vi "Save Cfg to GXML.vi"(8 "error in":errorcluster, 11 "Chassis Cfg":refnum<class "ChassisCfg.lvclass">) -> (0 "error out":errorcluster, 2 "GXML String":string="<GXML_Root>\r\n  <VoltGroup mems='3' id='Static Voltages'>\r\n    <GroupName type='String'>Static Voltages</GroupName>\r\n    <MeasType type='Enum U16' sel='Voltage'>0</MeasType>\r\n    <GroupMems dim='[33]' type='Cluster'>\r\n      <VoltChan mems='2'>\r\n        <ChanHdr mems='5'>\r\n          <ChanName type='String'>Mod4/ai0</ChanName>\r\n          <Alias type='String'></Alias>\r\n          <ModbusAddr type='String'>300047</ModbusAddr>\r\n          <Device type='String'>NI 9205</Device>\r\n          <ToModBus type='Bool'>TRUE</ToModBus>\r\n        </ChanHdr>\r\n        <VoltChanCfg mems='3'>\r\n          <VRange type='DBL'>10</VRange>\r\n          <Term_Cfg type='U16'>10083</Term_Cfg>\r\n          <Coupling type='U16'>10050</Coupling>\r\n        </VoltChanCfg>\r\n      </VoltChan>\r\n      <VoltChan mems='2'>\r\n        <ChanHdr mems='5'>\r\n          <ChanName type='String'>Mod4/ai1</ChanName>\r\n          <Alias type='String'></Alias>\r\n          <ModbusAddr type='String'>300049</ModbusAddr>\r\n          <Device type='String'>NI 9205</Device>\r\n          <ToModBus type='Bool'>TRUE</ToModBus>\r\n        </ChanHdr>\r\n        <VoltChanCfg mems='3'>\r\n          <VRange type='DBL'>10</VRange>\r\n          <Term_Cfg type='U16'>10083</Term_Cfg>\r\n          <Coupling type='U16'>10050</Coupling>\r\n        </VoltChanCfg>\r\n      </VoltChan>\r\n      <VoltChan mems='2'>\r\n        <ChanHdr mems='5'>\r\n          <ChanName type='String'>Mod4/ai2</ChanName>\r\n          <Alias type='String'></Alias>\r\n          <ModbusAddr type='String'>300051</ModbusAddr>\r\n          <Device type='String'>NI 9205</Device>\r\n          <ToModBus type='Bool'>TRUE</ToModBus>\r\n        </ChanHdr>\r\n        <VoltChanCfg mems='3'>\r\n          <VRange type='DBL'>10</VRange>\r\n          <Term_Cfg type='U16'>10083</Term_Cfg>\r\n          <Coupling type='U16'>10050</Coupling>\r\n        </VoltChanCfg>\r\n      </VoltChan>\r\n      <VoltChan mems='2'>\r\n        <ChanHdr mems='5'>\r\n          <ChanName type='String'>Mod4/ai3</ChanName>\r\n          <Alias type='String'></Alias>\r\n          <ModbusAddr type='String'>300053</ModbusAddr>\r\n          <Device type='String'>NI 9205</Device>\r\n          <ToModBus type='Bool'>TRUE</ToModBus>\r\n        </ChanHdr>\r\n        <VoltChanCfg mems='3'>\r\n          <VRange type='DBL'>10</VRange>\r\n          <Term_Cfg type='U16'>10083</Term_Cfg>\r\n          <Coupling type='U16'>10050</Coupling>\r\n        </VoltChanCfg>\r\n      </VoltChan>\r\n      <VoltChan mems='2'>\r\n        <ChanHdr mems='5'>\r\n          <ChanName type='String'>Mod4/ai4</ChanName>\r\n          <Alias type='String'></Alias>\r\n          <ModbusAddr type='String'>300055</ModbusAddr>\r\n          <Device type='String'>NI 9205</Device>\r\n          <ToModBus type='Bool'>TRUE</ToModBus>\r\n        </ChanHdr>\r\n        <VoltChanCfg mems='3'>\r\n          <VRange type='DBL'>10</VRange>\r\n          <Term_Cfg type='U16'>10083</Term_Cfg>\r\n          <Coupling type='U16'>10050</Coupling>\r\n        </VoltChanCfg>\r\n      </VoltChan>\r\n      <VoltChan mems='2'>\r\n        <ChanHdr mems='5'>\r\n          <ChanName type='String'>Mod4/ai5</ChanName>\r\n          <Alias type='String'></Alias>\r\n          <ModbusAddr type='String'>300057</ModbusAddr>\r\n          <Device type='String'>NI 9205</Device>\r\n          <ToModBus type='Bool'>TRUE</ToModBus>\r\n        </ChanHdr>\r\n        <VoltChanCfg mems='3'>\r\n          <VRange type='DBL'>10</VRange>\r\n          <Term_Cfg type='U16'>10083</Term_Cfg>\r\n          <Coupling type='U16'>10050</Coupling>\r\n        </VoltChanCfg>\r\n      </VoltChan>\r\n      <VoltChan mems='2'>\r\n        <ChanHdr mems='5'>\r\n          <ChanName type='String'>Mod4/ai6</ChanName>\r\n          <Alias type='String'></Alias>\r\n          <ModbusAddr type='String'>300059</ModbusAddr>\r\n          <Device type='String'>NI 9205</Device>\r\n          <ToModBus type='Bool'>TRUE</ToModBus>\r\n        </ChanHdr>\r\n        <VoltChanCfg mems='3'>\r\n          <VRange type='DBL'>10</VRange>\r\n          <Term_Cfg type='U16'>10083</Term_Cfg>\r\n          <Coupling type='U16'>10050</Coupling>\r\n        </VoltChanCfg>\r\n      </VoltChan>\r\n      <VoltChan mems='2'>\r\n        <ChanHdr mems='5'>\r\n          <ChanName type='String'>Mod4/ai7</ChanName>\r\n          <Alias type='String'></Alias>\r\n          <ModbusAddr type='String'>300061</ModbusAddr>\r\n          <Device type='String'>NI 9205</Device>\r\n          <ToModBus type='Bool'>TRUE</ToModBus>\r\n        </ChanHdr>\r\n        <VoltChanCfg mems='3'>\r\n          <VRange type='DBL'>10</VRange>\r\n          <Term_Cfg type='U16'>10083</Term_Cfg>\r\n          <Coupling type='U16'>10050</Coupling>\r\n        </VoltChanCfg>\r\n      </VoltChan>\r\n      <VoltChan mems='2'>\r\n        <ChanHdr mems='5'>\r\n          <ChanName type='String'>Mod4/ai8</ChanName>\r\n          <Alias type='String'></Alias>\r\n          <ModbusAddr type='String'>300063</ModbusAddr>\r\n          <Device type='String'>NI 9205</Device>\r\n          <ToModBus type='Bool'>TRUE</ToModBus>\r\n        </ChanHdr>\r\n        <VoltChanCfg mems='3'>\r\n          <VRange type='DBL'>10</VRange>\r\n          <Term_Cfg type='U16'>10083</Term_Cfg>\r\n          <Coupling type='U16'>10050</Coupling>\r\n        </VoltChanCfg>\r\n      </VoltChan>\r\n      <VoltChan mems='2'>\r\n        <ChanHdr mems='5'>\r\n          <ChanName type='String'>Mod4/ai9</ChanName>\r\n          <Alias type='String'></Alias>\r\n          <ModbusAddr type='String'>300065</ModbusAddr>\r\n          <Device type='String'>NI 9205</Device>\r\n          <ToModBus type='Bool'>TRUE</ToModBus>\r\n        </ChanHdr>\r\n        <VoltChanCfg mems='3'>\r\n          <VRange type='DBL'>10</VRange>\r\n          <Term_Cfg type='U16'>10083</Term_Cfg>\r\n          <Coupling type='U16'>10050</Coupling>\r\n        </VoltChanCfg>\r\n      </VoltChan>\r\n      <VoltChan mems='2'>\r\n        <ChanHdr mems='5'>\r\n          <ChanName type='String'>Mod4/ai10</ChanName>\r\n          <Alias type='String'></Alias>\r\n          <ModbusAddr type='String'>300067</ModbusAddr>\r\n          <Device type='String'>NI 9205</Device>\r\n          <ToModBus type='Bool'>TRUE</ToModBus>\r\n        </ChanHdr>\r\n        <VoltChanCfg mems='3'>\r\n          <VRange type='DBL'>10</VRange>\r\n          <Term_Cfg type='U16'>10083</Term_Cfg>\r\n          <Coupling type='U16'>10050</Coupling>\r\n        </VoltChanCfg>\r\n      </VoltChan>\r\n      <VoltChan mems='2'>\r\n        <ChanHdr mems='5'>\r\n          <ChanName type='String'>Mod4/ai11</ChanName>\r\n          <Alias type='String'></Alias>\r\n          <ModbusAddr type='String'>300069</ModbusAddr>\r\n          <Device type='String'>NI 9205</Device>\r\n          <ToModBus type='Bool'>TRUE</ToModBus>\r\n        </ChanHdr>\r\n        <VoltChanCfg mems='3'>\r\n          <VRange type='DBL'>10</VRange>\r\n          <Term_Cfg type='U16'>10083</Term_Cfg>\r\n          <Coupling type='U16'>10050</Coupling>\r\n        </VoltChanCfg>\r\n      </VoltChan>\r\n      <VoltChan mems='2'>\r\n        <ChanHdr mems='5'>\r\n          <ChanName type='String'>Mod4/ai12</ChanName>\r\n          <Alias type='String'></Alias>\r\n          <ModbusAddr type='String'>300071</ModbusAddr>\r\n          <Device type='String'>NI 9205</Device>\r\n          <ToModBus type='Bool'>TRUE</ToModBus>\r\n        </ChanHdr>\r\n        <VoltChanCfg mems='3'>\r\n          <VRange type='DBL'>10</VRange>\r\n          <Term_Cfg type='U16'>10083</Term_Cfg>\r\n          <Coupling type='U16'>10050</Coupling>\r\n        </VoltChanCfg>\r\n      </VoltChan>\r\n      <VoltChan mems='2'>\r\n        <ChanHdr mems='5'>\r\n          <ChanName type='String'>Mod4/ai13</ChanName>\r\n          <Alias type='String'></Alias>\r\n          <ModbusAddr type='String'>300073</ModbusAddr>\r\n          <Device type='String'>NI 9205</Device>\r\n          <ToModBus type='Bool'>TRUE</ToModBus>\r\n        </ChanHdr>\r\n        <VoltChanCfg mems='3'>\r\n          <VRange type='DBL'>10</VRange>\r\n          <Term_Cfg type='U16'>10083</Term_Cfg>\r\n          <Coupling type='U16'>10050</Coupling>\r\n        </VoltChanCfg>\r\n      </VoltChan>\r\n      <VoltChan mems='2'>\r\n        <ChanHdr mems='5'>\r\n          <ChanName type='String'>Mod4/ai14</ChanName>\r\n          <Alias type='String'></Alias>\r\n          <ModbusAddr type='String'>300075</ModbusAddr>\r\n          <Device type='String'>NI 9205</Device>\r\n          <ToModBus type='Bool'>TRUE</ToModBus>\r\n        </ChanHdr>\r\n        <VoltChanCfg mems='3'>\r\n          <VRange type='DBL'>10</VRange>\r\n          <Term_Cfg type='U16'>10083</Term_Cfg>\r\n          <Coupling type='U16'>10050</Coupling>\r\n        </VoltChanCfg>\r\n      </VoltChan>\r\n      <VoltChan mems='2'>\r\n        <ChanHdr mems='5'>\r\n          <ChanName type='String'>Mod4/ai15</ChanName>\r\n          <Alias type='String'></Alias>\r\n          <ModbusAddr type='String'>300077</ModbusAddr>\r\n          <Device type='String'>NI 9205</Device>\r\n          <ToModBus type='Bool'>TRUE</ToModBus>\r\n        </ChanHdr>\r\n        <VoltChanCfg mems='3'>\r\n          <VRange type='DBL'>10</VRange>\r\n          <Term_Cfg type='U16'>10083</Term_Cfg>\r\n          <Coupling type='U16'>10050</Coupling>\r\n        </VoltChanCfg>\r\n      </VoltChan>\r\n      <VoltChan mems='2'>\r\n        <ChanHdr mems='5'>\r\n          <ChanName type='String'>Mod4/ai16</ChanName>\r\n          <Alias type='String'></Alias>\r\n          <ModbusAddr type='String'>300079</ModbusAddr>\r\n          <Device type='String'>NI 9205</Device>\r\n          <ToModBus type='Bool'>TRUE</ToModBus>\r\n        </ChanHdr>\r\n        <VoltChanCfg mems='3'>\r\n          <VRange type='DBL'>10</VRange>\r\n          <Term_Cfg type='U16'>10083</Term_Cfg>\r\n          <Coupling type='U16'>10050</Coupling>\r\n        </VoltChanCfg>\r\n      </VoltChan>\r\n      <VoltChan mems='2'>\r\n        <ChanHdr mems='5'>\r\n          <ChanName type='String'>Mod4/ai17</ChanName>\r\n          <Alias type='String'></Alias>\r\n          <ModbusAddr type='String'>300081</ModbusAddr>\r\n          <Device type='String'>NI 9205</Device>\r\n          <ToModBus type='Bool'>TRUE</ToModBus>\r\n        </ChanHdr>\r\n        <VoltChanCfg mems='3'>\r\n          <VRange type='DBL'>10</VRange>\r\n          <Term_Cfg type='U16'>10083</Term_Cfg>\r\n          <Coupling type='U16'>10050</Coupling>\r\n        </VoltChanCfg>\r\n      </VoltChan>\r\n      <VoltChan mems='2'>\r\n        <ChanHdr mems='5'>\r\n          <ChanName type='String'>Mod4/ai18</ChanName>\r\n          <Alias type='String'></Alias>\r\n          <ModbusAddr type='String'>300083</ModbusAddr>\r\n          <Device type='String'>NI 9205</Device>\r\n          <ToModBus type='Bool'>TRUE</ToModBus>\r\n        </ChanHdr>\r\n        <VoltChanCfg mems='3'>\r\n          <VRange type='DBL'>10</VRange>\r\n          <Term_Cfg type='U16'>10083</Term_Cfg>\r\n          <Coupling type='U16'>10050</Coupling>\r\n        </VoltChanCfg>\r\n      </VoltChan>\r\n      <VoltChan mems='2'>\r\n        <ChanHdr mems='5'>\r\n          <ChanName type='String'>Mod4/ai19</ChanName>\r\n          <Alias type='String'></Alias>\r\n          <ModbusAddr type='String'>300085</ModbusAddr>\r\n          <Device type='String'>NI 9205</Device>\r\n          <ToModBus type='Bool'>TRUE</ToModBus>\r\n        </ChanHdr>\r\n        <VoltChanCfg mems='3'>\r\n          <VRange type='DBL'>10</VRange>\r\n          <Term_Cfg type='U16'>10083</Term_Cfg>\r\n          <Coupling type='U16'>10050</Coupling>\r\n        </VoltChanCfg>\r\n      </VoltChan>\r\n      <VoltChan mems='2'>\r\n        <ChanHdr mems='5'>\r\n          <ChanName type='String'>Mod4/ai20</ChanName>\r\n          <Alias type='String'></Alias>\r\n          <ModbusAddr type='String'>300087</ModbusAddr>\r\n          <Device type='String'>NI 9205</Device>\r\n          <ToModBus type='Bool'>TRUE</ToModBus>\r\n        </ChanHdr>\r\n        <VoltChanCfg mems='3'>\r\n          <VRange type='DBL'>10</VRange>\r\n          <Term_Cfg type='U16'>10083</Term_Cfg>\r\n          <Coupling type='U16'>10050</Coupling>\r\n        </VoltChanCfg>\r\n      </VoltChan>\r\n      <VoltChan mems='2'>\r\n        <ChanHdr mems='5'>\r\n          <ChanName type='String'>Mod4/ai21</ChanName>\r\n          <Alias type='String'></Alias>\r\n          <ModbusAddr type='String'>300089</ModbusAddr>\r\n          <Device type='String'>NI 9205</Device>\r\n          <ToModBus type='Bool'>TRUE</ToModBus>\r\n        </ChanHdr>\r\n        <VoltChanCfg mems='3'>\r\n          <VRange type='DBL'>10</VRange>\r\n          <Term_Cfg type='U16'>10083</Term_Cfg>\r\n          <Coupling type='U16'>10050</Coupling>\r\n        </VoltChanCfg>\r\n      </VoltChan>\r\n      <VoltChan mems='2'>\r\n        <ChanHdr mems='5'>\r\n          <ChanName type='String'>Mod4/ai22</ChanName>\r\n          <Alias type='String'></Alias>\r\n          <ModbusAddr type='String'>300091</ModbusAddr>\r\n          <Device type='String'>NI 9205</Device>\r\n          <ToModBus type='Bool'>TRUE</ToModBus>\r\n        </ChanHdr>\r\n        <VoltChanCfg mems='3'>\r\n          <VRange type='DBL'>10</VRange>\r\n          <Term_Cfg type='U16'>10083</Term_Cfg>\r\n          <Coupling type='U16'>10050</Coupling>\r\n        </VoltChanCfg>\r\n      </VoltChan>\r\n      <VoltChan mems='2'>\r\n        <ChanHdr mems='5'>\r\n          <ChanName type='String'>Mod4/ai23</ChanName>\r\n          <Alias type='String'></Alias>\r\n          <ModbusAddr type='String'>300093</ModbusAddr>\r\n          <Device type='String'>NI 9205</Device>\r\n          <ToModBus type='Bool'>TRUE</ToModBus>\r\n        </ChanHdr>\r\n        <VoltChanCfg mems='3'>\r\n          <VRange type='DBL'>10</VRange>\r\n          <Term_Cfg type='U16'>10083</Term_Cfg>\r\n          <Coupling type='U16'>10050</Coupling>\r\n        </VoltChanCfg>\r\n      </VoltChan>\r\n      <VoltChan mems='2'>\r\n        <ChanHdr mems='5'>\r\n          <ChanName type='String'>Mod4/ai24</ChanName>\r\n          <Alias type='String'></Alias>\r\n          <ModbusAddr type='String'>300095</ModbusAddr>\r\n          <Device type='String'>NI 9205</Device>\r\n          <ToModBus type='Bool'>TRUE</ToModBus>\r\n        </ChanHdr>\r\n        <VoltChanCfg mems='3'>\r\n          <VRange type='DBL'>10</VRange>\r\n          <Term_Cfg type='U16'>10083</Term_Cfg>\r\n          <Coupling type='U16'>10050</Coupling>\r\n        </VoltChanCfg>\r\n      </VoltChan>\r\n      <VoltChan mems='2'>\r\n        <ChanHdr mems='5'>\r\n          <ChanName type='String'>Mod4/ai25</ChanName>\r\n          <Alias type='String'></Alias>\r\n          <ModbusAddr type='String'>300097</ModbusAddr>\r\n          <Device type='String'>NI 9205</Device>\r\n          <ToModBus type='Bool'>TRUE</ToModBus>\r\n        </ChanHdr>\r\n        <VoltChanCfg mems='3'>\r\n          <VRange type='DBL'>10</VRange>\r\n          <Term_Cfg type='U16'>10083</Term_Cfg>\r\n          <Coupling type='U16'>10050</Coupling>\r\n        </VoltChanCfg>\r\n      </VoltChan>\r\n      <VoltChan mems='2'>\r\n        <ChanHdr mems='5'>\r\n          <ChanName type='String'>Mod4/ai26</ChanName>\r\n          <Alias type='String'></Alias>\r\n          <ModbusAddr type='String'>300099</ModbusAddr>\r\n          <Device type='String'>NI 9205</Device>\r\n          <ToModBus type='Bool'>TRUE</ToModBus>\r\n        </ChanHdr>\r\n        <VoltChanCfg mems='3'>\r\n          <VRange type='DBL'>10</VRange>\r\n          <Term_Cfg type='U16'>10083</Term_Cfg>\r\n          <Coupling type='U16'>10050</Coupling>\r\n        </VoltChanCfg>\r\n      </VoltChan>\r\n      <VoltChan mems='2'>\r\n        <ChanHdr mems='5'>\r\n          <ChanName type='String'>Mod4/ai27</ChanName>\r\n          <Alias type='String'></Alias>\r\n          <ModbusAddr type='String'>300101</ModbusAddr>\r\n          <Device type='String'>NI 9205</Device>\r\n          <ToModBus type='Bool'>TRUE</ToModBus>\r\n        </ChanHdr>\r\n        <VoltChanCfg mems='3'>\r\n          <VRange type='DBL'>10</VRange>\r\n          <Term_Cfg type='U16'>10083</Term_Cfg>\r\n          <Coupling type='U16'>10050</Coupling>\r\n        </VoltChanCfg>\r\n      </VoltChan>\r\n      <VoltChan mems='2'>\r\n        <ChanHdr mems='5'>\r\n          <ChanName type='String'>Mod4/ai28</ChanName>\r\n          <Alias type='String'></Alias>\r\n          <ModbusAddr type='String'>300103</ModbusAddr>\r\n          <Device type='String'>NI 9205</Device>\r\n          <ToModBus type='Bool'>TRUE</ToModBus>\r\n        </ChanHdr>\r\n        <VoltChanCfg mems='3'>\r\n          <VRange type='DBL'>10</VRange>\r\n          <Term_Cfg type='U16'>10083</Term_Cfg>\r\n          <Coupling type='U16'>10050</Coupling>\r\n        </VoltChanCfg>\r\n      </VoltChan>\r\n      <VoltChan mems='2'>\r\n        <ChanHdr mems='5'>\r\n          <ChanName type='String'>Mod4/ai29</ChanName>\r\n          <Alias type='String'></Alias>\r\n          <ModbusAddr type='String'>300105</ModbusAddr>\r\n          <Device type='String'>NI 9205</Device>\r\n          <ToModBus type='Bool'>TRUE</ToModBus>\r\n        </ChanHdr>\r\n        <VoltChanCfg mems='3'>\r\n          <VRange type='DBL'>10</VRange>\r\n          <Term_Cfg type='U16'>10083</Term_Cfg>\r\n          <Coupling type='U16'>10050</Coupling>\r\n        </VoltChanCfg>\r\n      </VoltChan>\r\n      <VoltChan mems='2'>\r\n        <ChanHdr mems='5'>\r\n          <ChanName type='String'>Mod4/ai30</ChanName>\r\n          <Alias type='String'></Alias>\r\n          <ModbusAddr type='String'>300107</ModbusAddr>\r\n          <Device type='String'>NI 9205</Device>\r\n          <ToModBus type='Bool'>TRUE</ToModBus>\r\n        </ChanHdr>\r\n        <VoltChanCfg mems='3'>\r\n          <VRange type='DBL'>10</VRange>\r\n          <Term_Cfg type='U16'>10083</Term_Cfg>\r\n          <Coupling type='U16'>10050</Coupling>\r\n        </VoltChanCfg>\r\n      </VoltChan>\r\n      <VoltChan mems='2'>\r\n        <ChanHdr mems='5'>\r\n          <ChanName type='String'>Mod4/ai31</ChanName>\r\n          <Alias type='String'></Alias>\r\n          <ModbusAddr type='String'>300109</ModbusAddr>\r\n          <Device type='String'>NI 9205</Device>\r\n          <ToModBus type='Bool'>TRUE</ToModBus>\r\n        </ChanHdr>\r\n        <VoltChanCfg mems='3'>\r\n          <VRange type='DBL'>10</VRange>\r\n          <Term_Cfg type='U16'>10083</Term_Cfg>\r\n          <Coupling type='U16'>10050</Coupling>\r\n        </VoltChanCfg>\r\n      </VoltChan>\r\n      <VoltChan mems='2'>\r\n        <ChanHdr mems='5'>\r\n          <ChanName type='String'>Mod6/ai3</ChanName>\r\n          <Alias type='String'></Alias>\r\n          <ModbusAddr type='String'>300111</ModbusAddr>\r\n          <Device type='String'>NI 9219</Device>\r\n          <ToModBus type='Bool'>TRUE</ToModBus>\r\n        </ChanHdr>\r\n        <VoltChanCfg mems='3'>\r\n          <VRange type='DBL'>60</VRange>\r\n          <Term_Cfg type='U16'>10106</Term_Cfg>\r\n          <Coupling type='U16'>10050</Coupling>\r\n        </VoltChanCfg>\r\n      </VoltChan>\r\n    </GroupMems>\r\n  </VoltGroup>\r\n</GXML_Root>")   [LabVIEW 2012, in "Configuration Grandmaster.lvlib" / "ChassisCfg.lvclass"]
uses:
  ChassisCfg.lvclass
  Custom Ctrls/Master CfgXML/ge_XMLHdr_TimingGrp.ctl
  Custom Ctrls/Master CfgXML/ge_XMLHdr_ChanGroups.ctl
  Custom Ctrls/Master Cfg/ge_GrpHdr.ctl
  Custom Ctrls/ge_MeasType.ctl
  ChassisCfg.lvclass/ChassisCfg.ctl
  Class Timing Group/Read Rate.vi
  Class Timing Group/Read ReadBlk.vi
  Class Timing Group/Read Modbus URL.vi
  Class Timing Group/Read ChanGroups.vi
  Class Chan Group/ChanGrp.lvclass
  Class Timing Group/TimingGrp.lvclass
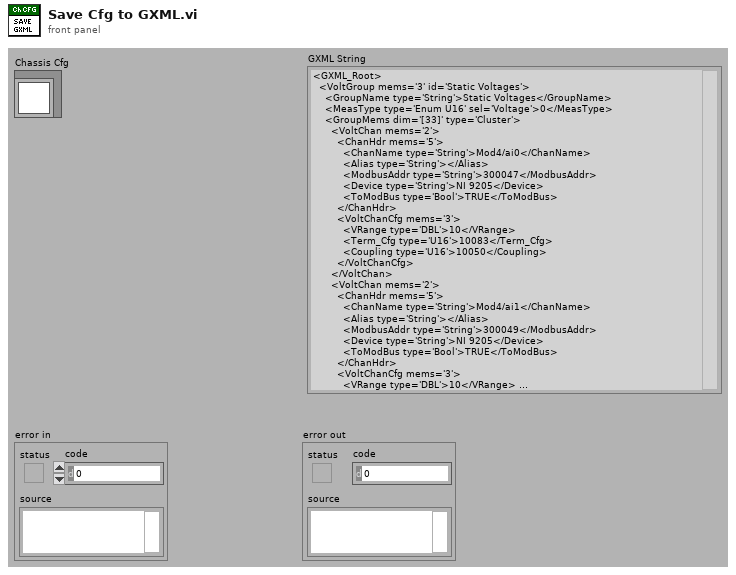
[diagram p1: front panel]
types:
  T1 = typedef "ge_XMLHdr_TimingGrp.ctl" = cluster{"Rate":dbl, "ReadBlk":i32, "Modbus URL":string, "ChanGroups":T2}
  T2 = typedef "ge_XMLHdr_ChanGroups.ctl" = T3[]
  T3 = typedef "ge_GrpHdr.ctl" = cluster{"GroupName":string, "MeasType":T4}
  T4 = typedef "ge_MeasType.ctl" = enum16{"Voltage", "Frequency", "Tachometer", "Dynamic", "Thermocouple", "RTD", "Strain", "Current", "Resistance"}
  T5 = typedef "LS Lock Sizes.ctl" = enum16{"No", "250ms", "500ms", "1s"}
  T6 = typedef "Chassis Type.ctl" = enum16{"Not Supported", "C Series 1-Slot", "C Series 4-Slot", "C Series 8-Slot", "PXI 8-Slot", "PXIe 18-Slot"}
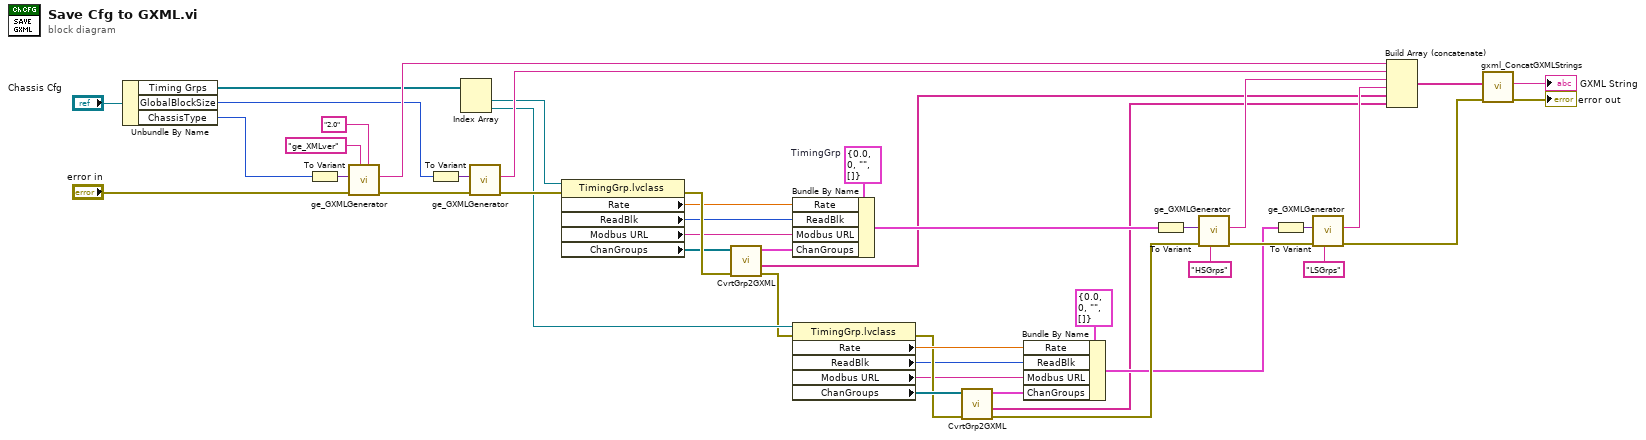
[diagram p0: block diagram]
diagram:
  w28 = T1 {"Rate"=0.0, "ReadBlk"=0, "Modbus URL"="", "ChanGroups"=[]}  # TimingGrp
  n1 = Unbundle By Name("Chassis Cfg") -> ("Timing Grps"=w32:refnum<class "TimingGrp.lvclass">[], "GlobalBlockSize"=w5:T5, "ChassisType"=w6:T6)
  n2 = To Variant(anything=w6) -> (Variant=w35:variant)
  n3 = call "ge_GXMLGenerator.vi"("Version String"="2.0", "Version Tag Name"="ge_XMLver", "error in"="error in", "Variant"=w35) -> ("error out"=w23:errorcluster, "XML String Out"=w41:string)  [unwired: 6 in]
  n4 = To Variant(anything=w5) -> (Variant=w34:variant)
  n5 = Index Array(array=w32) -> (element #1=w21:refnum<class "TimingGrp.lvclass">, element #2=w14:refnum<class "TimingGrp.lvclass">)  [unwired: 2 in]
  n6 = call "ge_GXMLGenerator.vi"("error in"=w23, "Variant"=w34) -> ("error out"=w22:errorcluster, "XML String Out"=w36:string)  [unwired: 8 in]
  n7 = property class="TimingGrp.lvclass"(reference=w21, error in=w22) -> (error out=w31:errorcluster, "Rate"=w25:dbl, "ReadBlk"=w2:i32, "Modbus URL"=w4:string, "ChanGroups"=w27:refnum<class "ChanGrp.lvclass">[])  [unwired: 1 out]
  n8 = call "CvrtGrp2GXML.vi"("error in (no error)"=w31, "ChanGroups in"=w27) -> ("error out"=w13:errorcluster, "GXML Chans Oout"=w11:string[], "ChanGroups out"=w26:T2)  [unwired: 7 in]
  n9 = Bundle By Name(cluster=w28, "Rate"=w25, "ReadBlk"=w2, "Modbus URL"=w4, "ChanGroups"=w26) -> (w24:T1)
  n10 = property class="TimingGrp.lvclass"(reference=w14, error in=w13) -> (error out=w15:errorcluster, "Rate"=w19:dbl, "ReadBlk"=w1:i32, "Modbus URL"=w3:string, "ChanGroups"=w17:refnum<class "ChanGrp.lvclass">[])  [unwired: 1 out]
  n11 = call "CvrtGrp2GXML.vi"("error in (no error)"=w15, "ChanGroups in"=w17) -> ("error out"=w12:errorcluster, "GXML Chans Oout"=w7:string[], "ChanGroups out"=w18:T2)  [unwired: 7 in]
  n12 = Bundle By Name(cluster=T1 {"Rate"=0.0, "ReadBlk"=0, "Modbus URL"="", "ChanGroups"=[]} ("TimingGrp"), "Rate"=w19, "ReadBlk"=w1, "Modbus URL"=w3, "ChanGroups"=w18) -> (w8:T1)
  n13 = To Variant(anything=w24) -> (Variant=w33:variant)
  n14 = call "ge_GXMLGenerator.vi"("String ID"="HSGrps", "error in"=w12, "Variant"=w33) -> ("error out"=w40:errorcluster, "XML String Out"=w42:string)  [unwired: 7 in]
  n15 = To Variant(anything=w8) -> (Variant=w9:variant)
  n16 = call "ge_GXMLGenerator.vi"("String ID"="LSGrps", "error in"=w40, "Variant"=w9) -> ("error out"=w29:errorcluster, "XML String Out"=w43:string)  [unwired: 7 in]
  n17 = Build Array (concatenate)(w41, w36, w42, w43, w11, w7) -> (w10:string[])
  n18 = call <userlib>:"gxml_ConcatGXMLStrings.vi"("error in"=w29, "GXML Strings"=w10) -> ("error out"=→"error out":errorcluster, "Concatenated GXML String"=→"GXML String":string)  [unwired: 8 in]
